vi "Unpack for gRPC.vi"(8 "error in":errorcluster, 9 "configuration / results":enum16{"Configuration", "Results"}(ring), 10 "any":T1, 11 "measurement plugin service in":refnum<class "Fake Measurement Plugin.lvclass">) -> (0 "error out":errorcluster, 2 "data value":variant, 3 "measurement plugin service in":refnum<class "Fake Measurement Plugin.lvclass">)   [LabVIEW 2020, in "MeasurementServerTests.lvlib" / "Measurement Plugin Service Tests.lvlib" / "Fake Measurement Plugin.lvclass"]
uses:
  Fake Measurement Plugin.lvclass
  <vilib>/gRPC/LabVIEW gRPC Library/Shared/Any.ctl
  <vilib>/MeasurementLink/MeasurementLink Measurement Server/Measurement Plugin Service/Measurement Plugin Service.lvclass
  <vilib>/gRPC/LabVIEW gRPC Library/grpc-lvsupport-release.lvlib
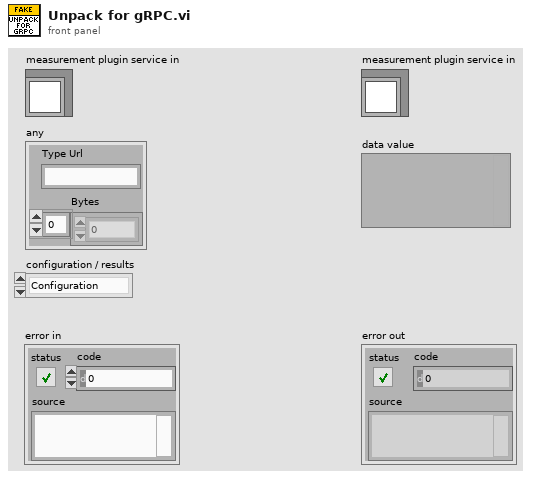
[diagram p1: front panel]
types:
  T1 = typedef "grpc-lvsupport-release.lvlib/Any.ctl" = cluster{"Type Url":string, "Bytes":u8[]}
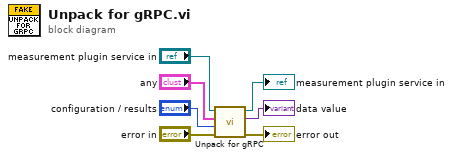
[diagram p0: block diagram]
diagram:
  n1 = call-parent "Unpack for gRPC.vi"("error in"="error in", "configuration / results"="configuration / results", "any"="any", "measurement plugin service in"="measurement plugin service in") -> ("error out"=→"error out":errorcluster, "data value"=→"data value":variant, "measurement plugin service out"=→"measurement plugin service in":refnum<class "Fake Measurement Plugin.lvclass">)  [unwired: 5 in]
